vi "Close All Net Use.vi"(8 "error in (no error)":errorcluster) -> (0 "error out":errorcluster)   [LabVIEW 2017, in "G3_Build Process File Utilities.lvlib"]
uses:
  G3_Build Process File Utilities.lvlib
panel:
  out "standard output":string
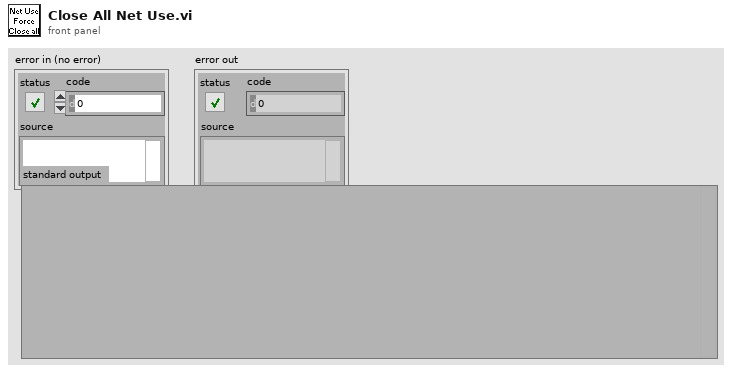
[diagram p1: front panel]
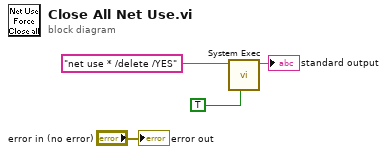
[diagram p0: block diagram]
diagram:
  n1 = call <vilib>:"System Exec.vi"("run minimized? (F)"=TRUE, "command line"="net use * /delete /YES") -> ("standard output"=→"standard output":string)  [unwired: 6 in, 3 out]
  "error out" <- "error in (no error)"
